vi "Modify Enqueue Data to Requested Node Size.vi"(7 "VI to Code Rel Path":string="IONode\\DLULayer\\Enqueue Data To Nodes.vi", 8 "Error In":errorcluster, 10 "NumCasesToAdd":i32=1, 11 "Source Root Path":path=path "C:/Users/kvemishe/Downloads/IONode/DLULayer/Enqueue Data To Nodes.vi") -> (0 "error out":errorcluster, 2 "Object Found?":bool, 3 "Source Root Path Out":path=path "C:/Users/kvemishe/Downloads/IONode/DLULayer/Enqueue Data To Nodes.vi")   [LabVIEW 2014]
doc: "This VI scripts the deque commands VI for the IO Node Engine"
uses:
  <vilib>/Utility/traverseref.llb/TRef TravTarget.ctl
  <vilib>/Utility/traverseref.llb/VI Scripting - Traverse.lvlib
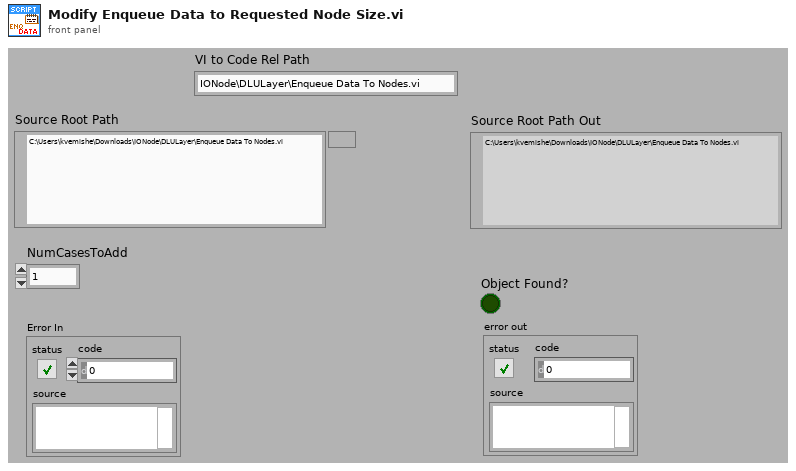
[diagram p1: front panel]
types:
  T1 = typedef "TRef TravTarget.ctl" = enum16{"FP", "BD", "Other"}
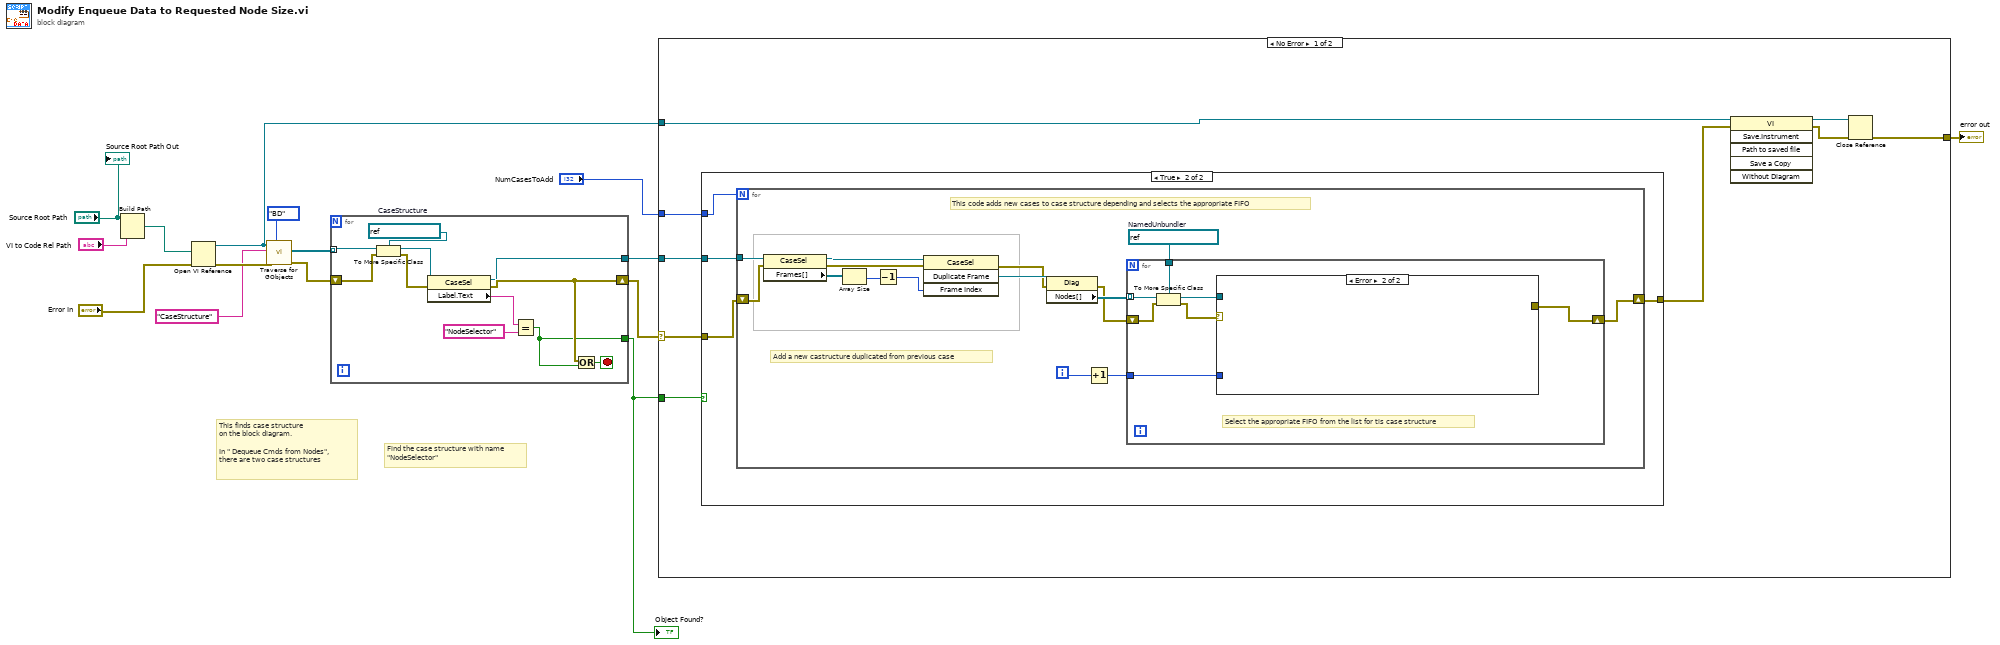
[diagram p0: block diagram]
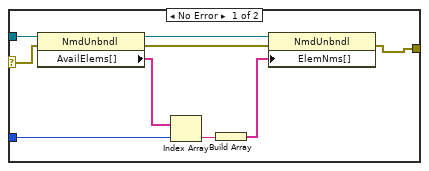
[diagram p3: hidden frame]
diagram:
  # "Find the case structure with name\n\"NodeSelector\""
  # "This finds case structure\non the block diagram.\n\nIn \" Dequeue Cmds from Nodes\",\nthere are two case structures"
  n1 = Build Path(base path="Source Root Path", name or relative path="VI to Code Rel Path") -> (appended path=w2:path)
  n2 = Open VI Reference(vi path=w2, error in (no error)="Error In") -> (vi reference=w6:refnum<vi>, error out=w14:errorcluster)  [unwired: 4 in]
  n3 = call <vilib>:"Traverse for GObjects.vi"("Traverse Target"=TRef_TravTarget."BD", "error in (no error)"=w14, "Class Name"="CaseStructure", "VI Refnum"=w6) -> ("error out"=w11:errorcluster, "References"=w12:refnum<vi>[])  [unwired: 4 in, 2 out]
  n4 = for {
    tunnel: w12 -> [w26] mode=indexing
    shift-right: [w18] -> w9
    shift-left: w11 -> [w24]
    tunnel: [w17] -> w8
    tunnel: [w16] -> w10
    stop <- w19 stop-if-true
    w25 = refnum<vi> refnum  # CaseStructure
    n5 = To More Specific Class(target class=w25, reference=w26, error in=w24) -> (specific class reference=w23:refnum<vi>, error out=w22:errorcluster)
    n6 = property class="CaseSel"(reference=w23, error in=w22) -> (reference out=w16:refnum<vi>, error out=w18:errorcluster, "Label.Text"=w21:string)
    n7 = Equal?(x=w21, y="NodeSelector") -> (x = y?=w17:bool)
    n8 = Or(x=w18, y=w17) -> (x .or. y?=w19:bool)
  }
  "Object Found?" <- w8
  n9 = case shown="No Error" w9 {
    selector: w9 -> [w32 w72]
    tunnel: w10 -> [w35 _]
    tunnel: w8 -> [w34 _]
    tunnel: "NumCasesToAdd" -> [w33 _]
    tunnel: w6 -> [w31 _]
    tunnel: [w27 w72] -> w4
    frame No Error {
      n10 = case shown="True" w34 {
        tunnel: w35 -> [_ w40]
        tunnel: w33 -> [_ w39]
        tunnel: w32 -> [w36 w37]
        tunnel: [w36 w38] -> w30
        frame False {
        }
        frame True {
          n11 = for {
            N: w39 -> [_]
            tunnel: w40 -> [w46]
            shift-right: [w41] -> w38
            shift-left: w37 -> [w42]
            i -> [w45]
            w48 = refnum<vi> refnum  # NamedUnbundler
            # "Add a new castructure duplicated from previous case"
            # "This code adds new cases to case structure depending and selects the appropriate FIFO"
            n12 = property class="CaseSel"(reference=w46, error in=w42) -> (reference out=w55:refnum<vi>, error out=w54:errorcluster, "Frames[]"=w53:refnum<vi>[])
            n13 = Array Size(array=w53) -> (size(s)=w52:i32)
            n14 = Decrement(x=w52) -> (x-1=w51:i32)
            n15 = invoke class="CaseSel" method="Duplicate Frame"(reference=w55, error in=w54, "Frame Index"=w51) -> (error out=w44:errorcluster, "Duplicate Frame"=w50:refnum<vi>)  [unwired: 1 in, 2 out]
            n16 = property class="Diag"(reference=w50, error in=w44) -> (error out=w43:errorcluster, "Nodes[]"=w49:refnum<vi>[])  [unwired: 1 out]
            n17 = Increment(x=w45) -> (x+1=w47:i32)
            n18 = for {
              tunnel: w49 -> [w62] mode=indexing
              tunnel: w48 -> [w61]
              tunnel: w47 -> [w58]
              shift-right: [w56] -> w41
              shift-left: w43 -> [w57]
              # "Select the appropriate FIFO from the list for tis case structure"
              n19 = To More Specific Class(target class=w61, reference=w62, error in=w57) -> (specific class reference=w59:refnum<vi>, error out=w60:errorcluster)
              n20 = case shown="Error" w60 {
                selector: w60 -> [w70 _]
                tunnel: w59 -> [w71 _]
                tunnel: w58 -> [w65 _]
                tunnel: [w63 _] -> w56
                frame No Error {
                  n21 = property class="NmdUnbndl"(reference=w71, error in=w70) -> (reference out=w69:refnum<vi>, error out=w64:errorcluster, "AvailElems[]"=w68:string[])
                  n22 = Index Array(array=w68, index=w65) -> (element=w67:string)
                  n23 = Build Array(w67) -> (w66:string[])
                  n24 = property class="NmdUnbndl"(reference=w69, error in=w64, "ElemNms[]"=w66) -> (error out=w63:errorcluster)  [unwired: 1 out]
                }
                frame Error {
                }
              }
            }
          }
        }
      }
      n25 = invoke class="VI" method="Save.Instrument"(reference=w31, error in=w30) -> (reference out=w29:refnum<vi>, error out=w28:errorcluster)  [unwired: 4 in, 4 out]
      n26 = Close Reference(reference=w29, error in (no error)=w28) -> (error out=w27:errorcluster)
    }
    frame Error {
    }
  }
  "error out" <- w4
  "Source Root Path Out" <- "Source Root Path"
